vi "8XYE.vi"(11 "Variables and Memory in":T1 {"GFX" format="%02x"}) -> (3 "Variables and Memory out":T1 {"GFX" format="%02x"})   [LabVIEW 2021]
uses:
  Controls/ClusterF.ctl
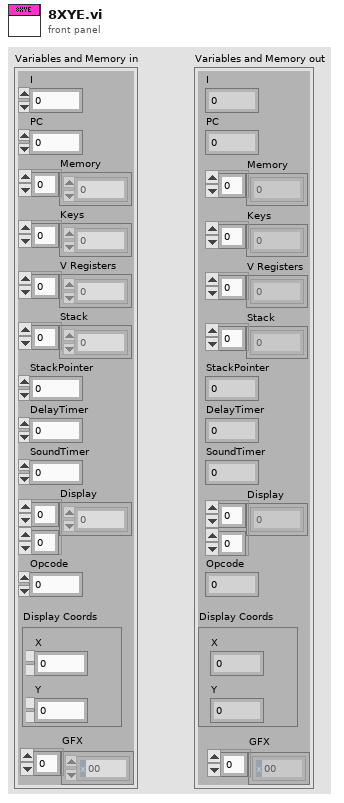
[diagram p1: front panel]
types:
  T1 = typedef "ClusterF.ctl" = cluster{"I":u16, "PC":u16, "Memory":u8[], "Keys":u8[], "V Registers":u8[], "Stack":u16[], "StackPointer":u16, "DelayTimer":u8, "SoundTimer":u8, "Display":u8[][], "Opcode":u16, "Display Coords":cluster{"X":u8, "Y":u8}, "GFX":u8[]}
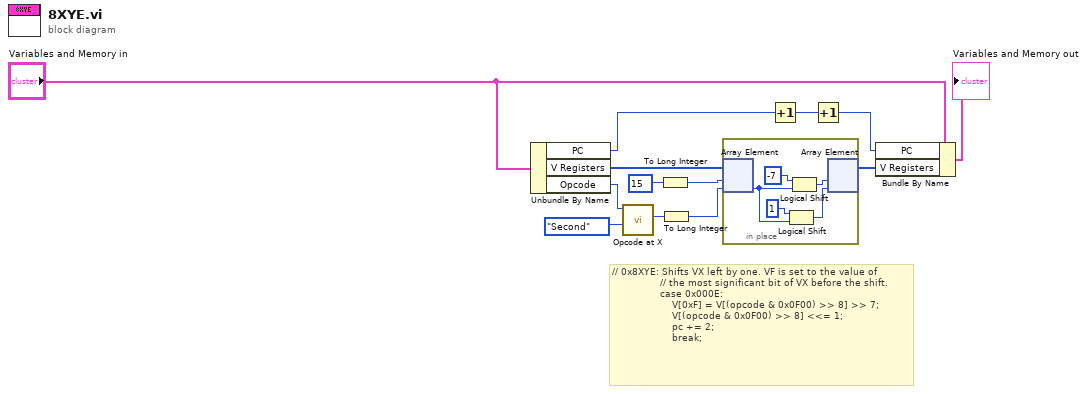
[diagram p0: block diagram]
diagram:
  # "// 0x8XYE: Shifts VX left by one. VF is set to the value of\n                // the most significant bit of VX before the shift.\n                case 0x000E:\n                    V[0xF] = V[(opcode & 0x0F00) >> 8] >> 7;\n                    V[(opcode & 0x0F00) >> 8] <<= 1;\n                    pc += 2;\n                    break;"
  n1 = Unbundle By Name("Variables and Memory in") -> ("PC"=w4:u16, "V Registers"=w8:u8[], "Opcode"=w6:u16)
  n2 = call "Opcode at X.vi"("X Position"=enum16{"First", "Second", "Third", "Fourth"}."Second", "Opcode"=w6) -> ("Opcode at X Position (U8)"=w11:u8)  [unwired: 9 in]
  n3 = To Long Integer(number=u8 15) -> (32bit integer=w10:i32)
  n4 = To Long Integer(number=w11) -> (32bit integer=w12:i32)
  n5 = in-place {
    n6 = in-place-array #1(w8, w10, w12) -> (w16:u8)  [unwired: 1 out]
    n7 = Logical Shift(y=i16 1, x=w16) -> (x << y=w14:u8)
    n8 = Logical Shift(y=i16 -7, x=w16) -> (x << y=w17:u8)
    n9 = in-place-array #1(w17, w14) -> (w13:u8[])  [unwired: 2 out]
  }
  n10 = Increment(x=w4) -> (x+1=w3:u16)
  n11 = Increment(x=w3) -> (x+1=w5:u16)
  n12 = Bundle By Name(cluster="Variables and Memory in", "PC"=w5, "V Registers"=w13) -> (→"Variables and Memory out":T1)
